vi "Write EDVR Pool.vi"(10 "DVR Pool":refnum<queue>, 11 "Template in":refnum<class "Template.lvclass">) -> (3 "Template out":refnum<class "Template.lvclass">)   [LabVIEW 2020, in "Template.lvlib" / "Template.lvclass"]
doc: "Sets the DVR Data queue reference"
uses:
  Template.lvclass
  Template.lvclass/Template.ctl
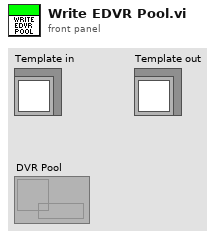
[diagram p1: front panel]
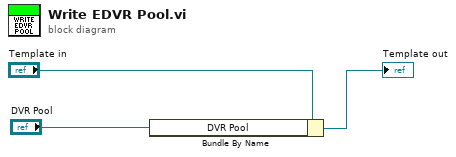
[diagram p0: block diagram]
diagram:
  n1 = Bundle By Name(cluster="Template in", "DVR Pool"="DVR Pool") -> (→"Template out":refnum<class "Template.lvclass">)
